vi "svfa_Compute Factors.vi"(1 "Number to be factored":i32) -> (0 "Factors of Input":i32[](array[numeric]))   [LabVIEW 2017]
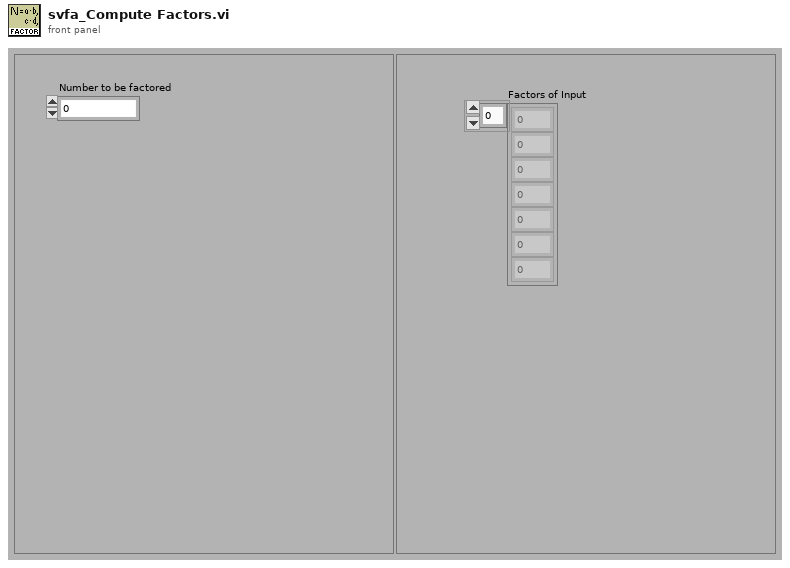
[diagram p1: front panel]
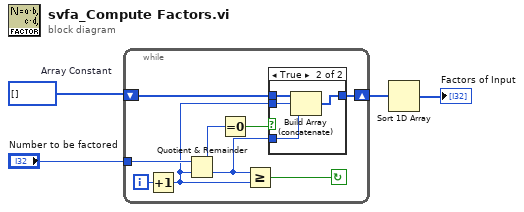
[diagram p0: block diagram]
diagram:
  w4 = i32[] []  # Array Constant
  n1 = while {
    shift-left: w4 -> [w9]
    shift-right: [w8] -> w2
    tunnel: "Number to be factored" -> [w13]
    i -> [w6]
    stop <- w12 continue-if-true
    n2 = Increment(x=w6) -> (x+1=w5:i32)
    n3 = Quotient & Remainder(x=w13, y=w5) -> (x-y*floor(x/y)=w11:i32, floor(x/y)=w7:i32)
    n4 = Equal To 0?(x=w11) -> (x = 0?=w10:bool)
    n5 = Greater Or Equal?(x=w7, y=w5) -> (x >= y?=w12:bool)
    n6 = case shown="True" w10 {
      tunnel: w9 -> [w14 w18]
      tunnel: w5 -> [_ w17]
      tunnel: [w14 w16] -> w8
      tunnel: w7 -> [_ w15]
      frame False {
      }
      frame True {
        n7 = Build Array (concatenate)(w18, w17, w15) -> (w16:i32[])
      }
    }
  }
  n8 = Sort 1D Array(array=w2) -> (sorted array=→"Factors of Input":i32[])
